vi "test.vi"() -> ()   [LabVIEW 2015]
uses:
  Container/Container.lvclass
  A/A.lvclass
  Parent/Parent.lvclass
  B/B.lvclass
panel:
  out "error out":errorcluster caption="sortie d'erreur"
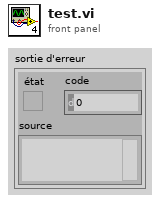
[diagram p1: front panel]
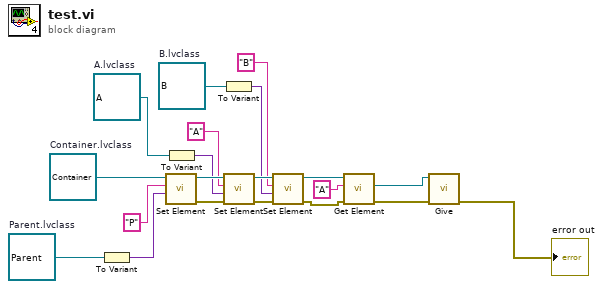
[diagram p0: block diagram]
diagram:
  w11 = refnum<class "B.lvclass"> refnum  # B.lvclass
  w5 = refnum<class "Parent.lvclass"> refnum  # Parent.lvclass
  w13 = refnum<class "A.lvclass"> refnum  # A.lvclass
  w8 = refnum<class "Container.lvclass"> refnum  # Container.lvclass
  n1 = To Variant(anything=w5) -> (Variant=w14:variant)
  n2 = call "Set Element.vi"("variant"=w14, "nom"="P", "Container en entrée"=w8) -> ("error out"=w18:errorcluster, "Container en sortie"=w19:refnum<class "Container.lvclass">)  [unwired: 7 in]
  n3 = To Variant(anything=w13) -> (Variant=w12:variant)
  n4 = To Variant(anything=w11) -> (Variant=w10:variant)
  n5 = call "Set Element.vi"("error in (no error)"=w18, "variant"=w12, "nom"="A", "Container en entrée"=w19) -> ("error out"=w15:errorcluster, "Container en sortie"=w16:refnum<class "Container.lvclass">)  [unwired: 6 in]
  n6 = call "Set Element.vi"("error in (no error)"=w15, "variant"=w10, "nom"="B", "Container en entrée"=w16) -> ("error out"=w3:errorcluster, "Container en sortie"=w7:refnum<class "Container.lvclass">)  [unwired: 6 in]
  n7 = call "Get Element.vi"("error in (no error)"=w3, "nom"="A", "Container en entrée"=w7) -> ("error out"=w1:errorcluster, "données"=w2:refnum<class "Parent.lvclass">)  [unwired: 6 in, 1 out]
  n8 = call-dynamic "Give.vi"("error in (no error)"=w1, "Parent en entrée"=w2) -> ("error out"=→"error out":errorcluster)  [unwired: 8 in, 1 out]
